vi "Camera Calibration Example.vi"() -> ()   [LabVIEW 2025]
uses:
  <vilib>/Rock Robotics/WPI/Camera/WPI_CameraSettings Read MJPG.ctl
  <vilib>/Rock Robotics/WPI/Camera/WPI_CameraImageSize.ctl
  <vilib>/Rock Robotics/WPI/Camera/WPI_CameraExposure Values.ctl
  <vilib>/Rock Robotics/WPI/Camera/WPI_CameraWhite Balance Values.ctl
  <vilib>/vision/NI_Vision_Development_Module.lvlib
panel:
  in  "File Path":path=path "File Path"
  in  "Camera Settings":T1={"fps"=20, "compression"=30, "Image Size"=enum."320x240", "Config Shown"=FALSE}
  in  "Camera Address":string="USB 1"
  in  "Camera Settings 2":T5={"Exposure"=enum."Auto", "Exposure (%)"=50.0, "Brightness"=50, "White Balance"=enum."Auto", "Color Temp (K)"=0.0} {"Brightness" min=0 max=100}
  out "Instructions:":string="Use the File Path to load image files from a directory, or use a USB or IP camera connected to your laptop. Use Camera Settings 1 and 2 to achieve a dark image with bright and colorful stripes.\nLED Color can encoded as HSL or related color modes. Calibrate to the same color as the strips being reflected to the camera.\nClick and draw a line in Original Image to auto-calibrate the LED Color. You may want to widen and tweak Sat and Val by hand.\n\nThere are lots of comments on the diagram to explain the code."
  in  "Color Mode":u16(ring)=2 items=["RGB", "HSL", "HSV", "HSI"]
  in  "Std Devs for Cal":cluster{"H":dbl, "S":dbl, "V":dbl}={"H"=4.0, "S"=6.0, "V"=6.0}
  in  "LED Color":T6={"Hue"={107.81818389892578, 139.81818389892578}, "Sat"={176.07142857142858, 255.0}, "Val"={40.53571428571429, 255.0}} {"Hue" scale=0.0..255.0 scale format="%#_3g"}
  out "Original Image":T7(plugin-control)
  out "LED Masked image":T7(plugin-control)
  out "RGBs of LED masked Pixels":u32[][](graph)
  out "V":u32[](graph)
  out "S":u32[](graph)
  out "Complete Image Histograms":u32[](graph)
  # "Top three graphs are typically the Hue, Saturation, and\nValue. Value is most helpful to show the \"darkness\" of\nthe majority of pixels.  If you change the color mode, the\ncomponents shown in the graph will be the requested\nelements."
  # "The next two displays are the masked image, using the LED\nColor, and the RGB components of the masked area -- to\nverify that none of the channels are saturated for a colored\nlight."
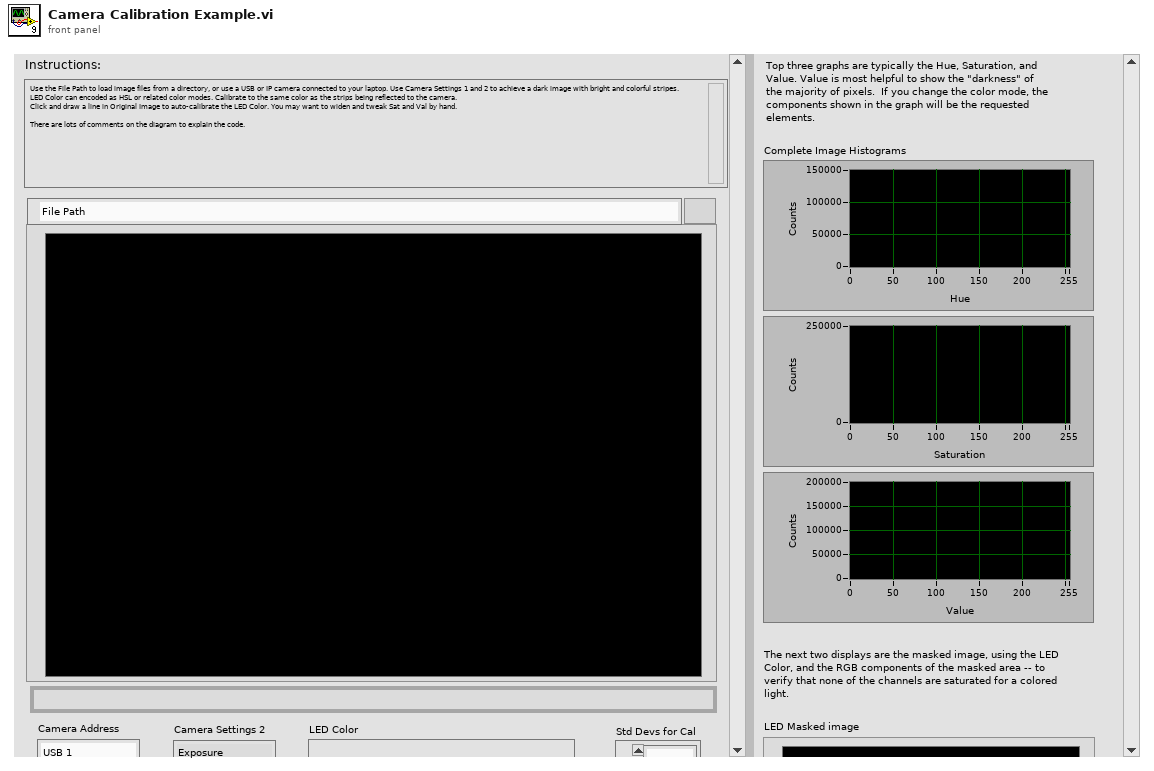
[diagram p1: front panel]
types:
  T1 = typedef "WPI_CameraSettings Read MJPG.ctl" = cluster{"fps":i32, "compression":i32, "Image Size":T2, "Config Shown":bool}
  T2 = typedef "WPI_CameraImageSize.ctl" = enum16{"640x480", "320x240", "160x120", "Custom"}
  T3 = typedef "WPI_CameraExposure Values.ctl" = enum16{"Auto", "Flicker-free 50 Hz", "Flicker-free 60 Hz", "Hold current", "Custom"}
  T4 = typedef "WPI_CameraWhite Balance Values.ctl" = enum16{"Auto", "Fixed indoor", "Fixed outdoor 1", "Fixed outdoor 2", "Fixed fluorescent 1", "Fixed fluorescent 2", "Hold current", "Custom"}
  T5 = cluster{"Exposure":T3, "Exposure (%)":dbl, "Brightness":i32, "White Balance":T4, "Color Temp (K)":dbl}
  T6 = cluster{"Hue":cluster{dbl, dbl}, "Sat":cluster{dbl, dbl}, "Val":cluster{dbl, dbl}}
  T7 = typedef "IMAQ Image.ctl" = refnum<image>
  T8 = typedef "Image Type" = u32
  T9 = cluster{cluster{dbl, dbl}, cluster{dbl, dbl}, cluster{dbl, dbl}}
  T10 = cluster{"histogram":u32[], "Minimal Value":sgl, "Maximal Value":sgl, "Starting Value":sgl, "Interval Width":sgl, "Mean Value":sgl, "Standard  Variation":sgl, "Area (pixels)":i32}
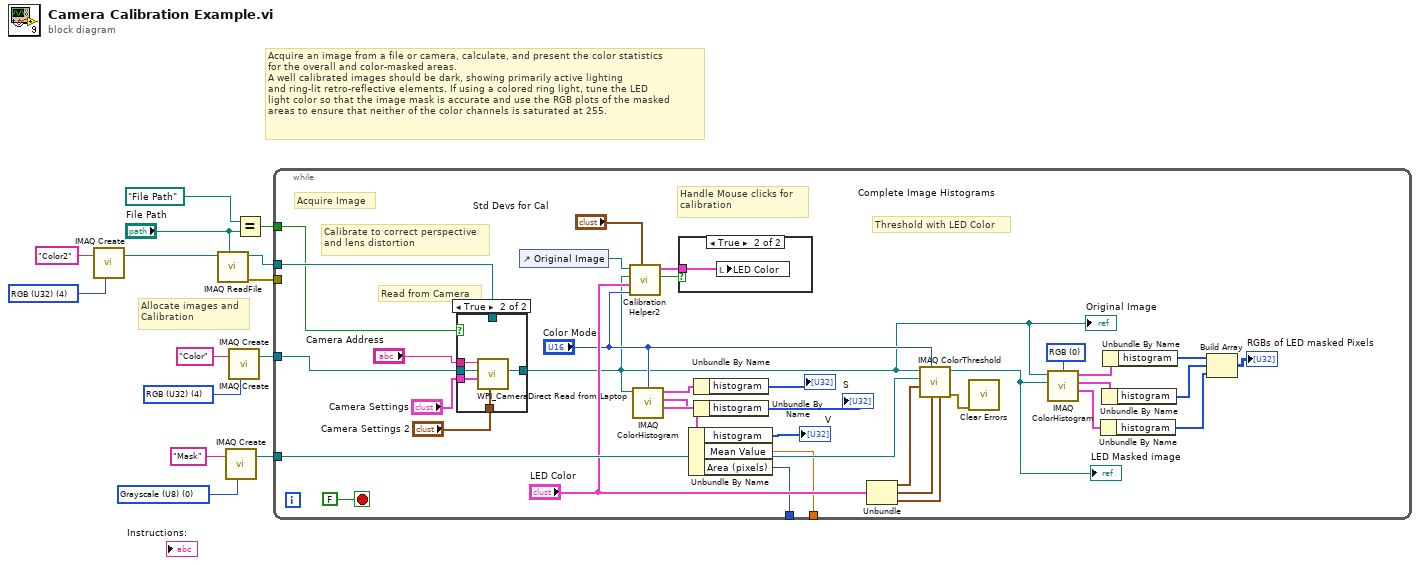
[diagram p0: block diagram]
diagram:
  w7 = T8 4 items=["Grayscale (U8)", "Grayscale (I16)", "Grayscale (SGL)", "Complex (CSG)", "RGB (U32)", "HSL (U32)", "RGB (U64)", "Grayscale (U16)"] ("Image Type")
  w10 = T8 4 items=["Grayscale (U8)", "Grayscale (I16)", "Grayscale (SGL)", "Complex (CSG)", "RGB (U32)", "HSL (U32)", "RGB (U64)", "Grayscale (U16)"] ("Image Type")
  w14 = T8 0 items=["Grayscale (U8)", "Grayscale (I16)", "Grayscale (SGL)", "Complex (CSG)", "RGB (U32)", "HSL (U32)", "RGB (U64)", "Grayscale (U16)"] ("Image Type")
  w15 = T8 4 items=["Grayscale (U8)", "Grayscale (I16)", "Grayscale (SGL)", "Complex (CSG)", "RGB (U32)", "HSL (U32)", "RGB (U64)", "Grayscale (U16)"] ("Image Type")
  # "Acquire an image from a file or camera, calculate, and present the color statistics\nfor the overall and color-masked areas.\nA well calibrated images should be dark, showing primarily active lighting\nand ring-lit retro-reflective elements. If using a colored ring light, tune the LED\nlight color so that the image mask is accurate and use the RGB plots of the masked\nareas to ensure that neither of the color channels is saturated at 255."
  # "Allocate images and\nCalibration"
  n1 = call "IMAQ Create"("Image Name"="Color2", "Image Type"=w7) -> ("New Image"=w6:T7)  [unwired: 2 in, 2 out]
  n2 = call "IMAQ ReadFile"("File Path"="File Path", "Image"=w6) -> ("error out"=w1:errorcluster, "Image Out"=w5:T7)  [unwired: 5 in, 3 out]
  n3 = call "IMAQ Create"("Image Name"="Mask", "Image Type"=w14) -> ("New Image"=w12:T7)  [unwired: 2 in, 2 out]
  n4 = call "IMAQ Create"("Image Name"="Color", "Image Type"=w10) -> ()  [unwired: 2 in, 3 out]
  n5 = call "IMAQ Create"("Image Name"="Color", "Image Type"=w15) -> ("New Image"=w11:T7)  [unwired: 2 in, 2 out]
  n6 = Equal?(x=path "File Path" ("File Path"), y="File Path") -> (x = y?=w3:bool)
  n7 = while {
    tunnel: w11 -> [w52]
    tunnel: w12 -> [w50]
    tunnel: [w30] -> _
    tunnel: w5 -> [w25]
    tunnel: [w23] -> _
    tunnel: w3 -> [w17]
    tunnel: w1 -> [_]
    stop <- FALSE stop-if-true
    w24 = u16 0 items=["RGB", "HSL", "HSV", "HSI", "CIE L*a*b*", "CIE XYZ"] ("Color Mode")
    # "Read from Camera"
    # "Calibrate to correct perspective\nand lens distortion"
    # "Handle Mouse clicks for\ncalibration"
    # "Threshold with LED Color"
    # "Acquire Image"
    n8 = case shown="True" w17 {
      tunnel: w52 -> [_ w58]
      tunnel: "Camera Address" -> [_ w57]
      tunnel: "Camera Settings" -> [_ w56]
      tunnel: "Camera Settings 2" -> [_ w55]
      tunnel: [w53 w54] -> w29
      tunnel: w25 -> [w53 _]
      frame False {
      }
      frame True {
        n9 = call <vilib>:"WPI_CameraDirect Read from Laptop.vi"("Camera Settings 2"=w55, "Camera Settings"=w56, "Image"=w58, "address"=w57) -> ("Image Out"=w54:T7)  [unwired: 6 in, 1 out]
      }
    }
    "Original Image" <- w29
    n10 = control-ref of="Original Image"() -> (w45:refnum<vi>)
    n11 = call "Calibration Helper2.vi"("Std Devs"="Std Devs for Cal", "Color Mode"="Color Mode", "Color Components"="LED Color", "Image"=w29, "Image Ctl Refnum"=w45) -> ("Changed"=w44:bool, "output color"=w43:T9)  [unwired: 5 in]
    n12 = call "IMAQ ColorHistogram"("Color Mode"="Color Mode", "Image Src"=w29) -> ("Red or Hue or X or L* Histogram Report"=w34:T10, "Green or Sat or Y or a* Histogram Report"=w35:T10, "Blue or Luma or Val or Inten or Z or b* Histogram Report"=w36:T10)  [unwired: 4 in, 1 out]
    n13 = case shown="True" w44 {
      tunnel: w43 -> [_ w59]
      frame False {
      }
      frame True {
        n14 = local write "LED Color"(w59) -> ()
      }
    }
    n15 = Unbundle By Name(w36) -> ("histogram"=→"V":u32[], "Mean Value"=w30:sgl, "Area (pixels)"=w23:i32)
    n16 = Unbundle By Name(w34) -> ("histogram"=→"Complete Image Histograms":u32[])
    n17 = Unbundle By Name(w35) -> ("histogram"=→"S":u32[])
    n18 = Unbundle("LED Color") -> ("Hue"=w49:cluster{dbl, dbl}, "Sat"=w48:cluster{dbl, dbl}, "Val"=w47:cluster{dbl, dbl})
    n19 = call "IMAQ ColorThreshold"("Blue or Luma or Val or Inten Range"=w47, "Green or Sat Range"=w48, "Color Mode"="Color Mode", "Red or Hue Range"=w49, "Image Dst"=w50, "Image Src"=w29) -> ("error out"=w46:errorcluster, "Image Dst Out"=w18:T7)  [unwired: 4 in]
    "LED Masked image" <- w18
    n20 = call <vilib>:"Clear Errors.vi"("error in (no error)"=w46) -> ()  [unwired: 5 in, 2 out]
    n21 = call "IMAQ ColorHistogram"("Color Mode"=w24, "Image Src"=w29, "Image Mask"=w18) -> ("Red or Hue or X or L* Histogram Report"=w28:T10, "Green or Sat or Y or a* Histogram Report"=w26:T10, "Blue or Luma or Val or Inten or Z or b* Histogram Report"=w27:T10)  [unwired: 3 in, 1 out]
    n22 = Unbundle By Name(w27) -> ("histogram"=w20:u32[])
    n23 = Unbundle By Name(w26) -> ("histogram"=w21:u32[])
    n24 = Unbundle By Name(w28) -> ("histogram"=w22:u32[])
    n25 = Build Array(w22, w21, w20) -> (→"RGBs of LED masked Pixels":u32[][])
  }
